vi "New JSON ({Value}).vi"(7 "key":string, 8 "error in (no error)":errorcluster, 10 "JSON Value in":refnum<class "JSON Value.lvclass">) -> (0 "error out":errorcluster, 3 "JSON Value out":refnum<class "JSON Value.lvclass">)   [LabVIEW 2016, in "JSON Value.lvclass"]
doc: "Create a new JSON Object initialized with the given key value pair."
uses:
  JSON Value.lvclass
  Object/Insert Value/Insert Value (Value).vi
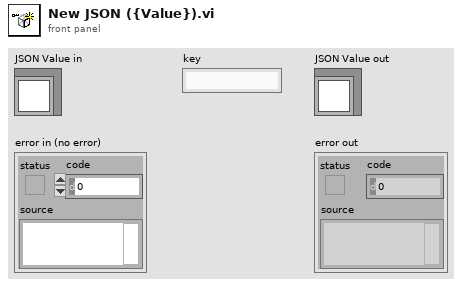
[diagram p1: front panel]
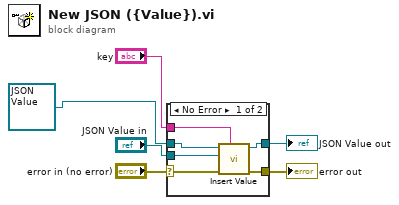
[diagram p0: block diagram]
diagram:
  n1 = case shown="No Error" "error in (no error)" {
    selector: "error in (no error)" -> [w12 w14]
    tunnel: [w11 w14] -> w5
    tunnel: [w9 w13] -> w4
    tunnel: refnum<class "JSON Value.lvclass"> refnum ("JSON out") -> [w10 w13]
    tunnel: "key" -> [w8 _]
    tunnel: "JSON Value in" -> [w7 _]
    frame No Error {
      n2 = call-poly "Insert Value.vi"("key"=w8, "error in (no error)"=w12, 10:"JSON Value in"=w7, 11:"JSON Value in"=w10) -> ("error out"=w11:errorcluster, "JSON Value out"=w9:refnum<class "JSON Value.lvclass">)  [unwired: 5 in, 1 out]
    }
    frame Error {
    }
  }
  "error out" <- w5
  "JSON Value out" <- w4
